vi "is_path.vi"(11 "data in":string) -> (1 "confirmed?":bool, 3 "data out":variant)   [LabVIEW 2020, in "configuration-data.lvclass"]
uses:
  configuration-data.lvclass
  <vilib>/regexp/Match Regular Expression.xnode
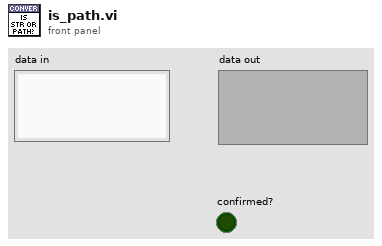
[diagram p1: front panel]
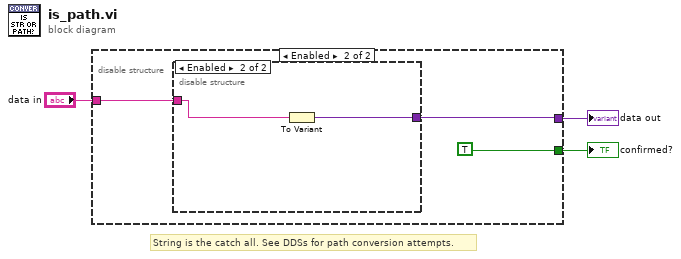
[diagram p0: block diagram]
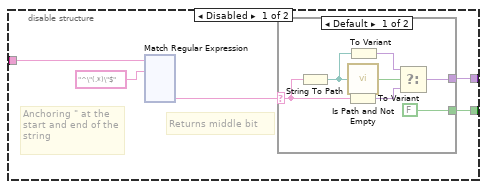
[diagram p2: hidden frame]
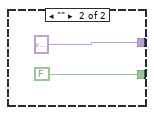
[diagram p3: hidden frame]
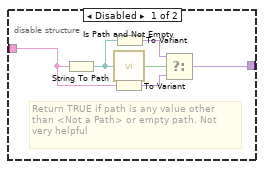
[diagram p4: hidden frame]
diagram:
  # "String is the catch all. See DDSs for path conversion attempts."
  n1 = disable-structure shown="Enabled" {
    disable-tunnel: [w8 TRUE] -> w3
    disable-tunnel: "data in" -> [w6 w134]
    disable-tunnel: [w4 w136] -> w1
    frame Disabled {
      # "Returns middle bit"
      # "Anchoring \" at the start and end of the string"
      n2 = xnode "Match Regular Expression"("input string"=w6, "regular expression"="^\"(.*)\"$") -> ("submatch 1"=w5:string)  [unwired: 4 in, 5 out]
      n3 = case shown="Default" w5 {
        selector: w5 -> [w129 _]
        tunnel: [FALSE FALSE] -> w8
        tunnel: [w125 variant] -> w4
        frame Default {
          n4 = String To Path(string=w129) -> (path=w130:path)
          n5 = call <vilib>:"Is Path and Not Empty.vi"("path"=w130) -> ("Is Path and Not Empty?"=w128:bool)  [unwired: 4 in]
          n6 = To Variant(anything=w129) -> (Variant=w126:variant)
          n7 = To Variant(anything=w130) -> (Variant=w127:variant)
          n8 = Select(t=w127, s=w128, f=w126) -> (s? t:f=w125:variant)
        }
        frame "" {
        }
      }
    }
    frame Enabled {
      n9 = disable-structure shown="Enabled" {
        disable-tunnel: [w138 w143] -> w136
        disable-tunnel: w134 -> [w137 w144]
        frame Disabled {
          # "Return TRUE if path is any value other than <Not a Path> or empty path. Not very helpful"
          n10 = String To Path(string=w137) -> (path=w142:path)
          n11 = call <vilib>:"Is Path and Not Empty.vi"("path"=w142) -> ("Is Path and Not Empty?"=w141:bool)  [unwired: 4 in]
          n12 = To Variant(anything=w137) -> (Variant=w139:variant)
          n13 = To Variant(anything=w142) -> (Variant=w140:variant)
          n14 = Select(t=w140, s=w141, f=w139) -> (s? t:f=w138:variant)
        }
        frame Enabled {
          n15 = To Variant(anything=w144) -> (Variant=w143:variant)
        }
      }
    }
  }
  "confirmed?" <- w3
  "data out" <- w1
